vi "DisplacementTest.vi"() -> ()   [LabVIEW 2016]
uses:
  Displacement/DisplacementErrorCodes.ctl
  Telemetry/TelemetryFields.ctl
  <vilib>/rvi/Emulation/niFpgaGetClockAttributes.vi
  <vilib>/rvi/Emulation/niFpgaSctlEmulationGetInTimedLoop.vi
  <vilib>/rvi/Emulation/niFpgaEmulationReportErrorSimple.vi
  <vilib>/rvi/Emulation/niFpgaEmulationIsFPGAContextNoSignature.vi
  <vilib>/rvi/errors/niFpgaSetErrorForExecOnDevCompSimple.vi
  <vilib>/rvi/eio/common/nirviEmuReportErrorAndStop.vi
  <vilib>/rvi/DataTransferAndStorage/Container/Common/niFpgaContainerGetUniqueNameForEmu.vi
  <vilib>/rvi/FIFO/Fifo_Resource/nirvififoEmulationSetSize.vi
  <vilib>/rvi/FIFO/Fifo_Resource/nirviFifoEmulationQueueMgr.vi
  <instcachedir>/0/nirviFifoEmulationQueueMgr_E5CAEC123FF24DC58D834DCA3CDAA9B5.lvgen/nirviFifoEmulationQueueMgr_E5CAEC123FF24DC58D834DCA3CDAA9B5_004.vi
  <vilib>/rvi/FIFO/Fifo_Resource/nirvififoEmulationDetermineInputValidOut.vi
  <vilib>/rvi/FIFO/Fifo_Resource/nirvififoEmulationCreateLock.vi
  <vilib>/rvi/Emulation/niFpgaProcessEmulError.vi
  <vilib>/rvi/FIFO/Fifo_Resource/nirvififoEmulationObtainLock.vi
  <vilib>/rvi/FIFO/Fifo_Resource/nirvififoEmulationReleaseLock.vi
  <vilib>/rvi/occurrence/nirviWaitOnOccurrenceBase.vi
  <vilib>/rvi/errors/nirviReportUnexpectedCaseInternalError.vi
  <vilib>/rvi/errors/nirviReportUnexpectedCaseInternalError (U32).vi
  <vilib>/Utility/error.llb/Clear Errors.vi
  <vilib>/rvi/Emulation/niFpgaCriticalErrorInLSC.vi
  <vilib>/rvi/Memory/Memory_Emulation/nirvimemoryFastEmulation.vi
  <vilib>/rvi/Memory/Memory_Emulation/nirvimemoryEmulation.vi
  <vilib>/rvi/DataTransferAndStorage/Container/Common/niFpgaContainerExecOnDevCompGetState.vi
  <vilib>/rvi/Memory/Memory_Emulation/niFpgaMemoryEmulationCacheClearOnFirstRun.vi
  <vilib>/rvi/Memory/Memory_Emulation/nirvimemoryEmulationManagerCache_MakeExclusive.vi
  <vilib>/rvi/Memory/Memory_Emulation/niFpgaMemoryEmulationValidateCache.vi
  <vilib>/rvi/Memory/Memory_Emulation/nirvimemoryEmulationManagerCache_InsertValue.vi
  <vilib>/rvi/Memory/Memory_Emulation/nirvimemoryEmulationManagerCache_ReleaseExclusive.vi
  <vilib>/rvi/Memory/Memory_Emulation/nirvimemoryEmulationManagerCache_GetValue.vi
  <vilib>/rvi/Memory/Memory_Emulation/nirvimemoryEmulationManagerCache_SetValue.vi
  <vilib>/rvi/Emulation/niFpgaSctlEmulationResourceMgr.vi
  <instcachedir>/0/nirviFifoEmulationQueueMgr_E5CAEC123FF24DC58D834DCA3CDAA9B5.lvgen/nirviFifoEmulationQueueMgr_E5CAEC123FF24DC58D834DCA3CDAA9B5_035.vi
  <instcachedir>/0/nirviFifoEmulationQueueMgr_E5CAEC123FF24DC58D834DCA3CDAA9B5.lvgen/nirviFifoEmulationQueueMgr_E5CAEC123FF24DC58D834DCA3CDAA9B5_033.vi
  <instcachedir>/0/nirviFifoEmulationQueueMgr_E5CAEC123FF24DC58D834DCA3CDAA9B5.lvgen/nirviFifoEmulationQueueMgr_E5CAEC123FF24DC58D834DCA3CDAA9B5_030.vi
  <instcachedir>/0/nirviFifoEmulationQueueMgr_E5CAEC123FF24DC58D834DCA3CDAA9B5.lvgen/nirviFifoEmulationQueueMgr_E5CAEC123FF24DC58D834DCA3CDAA9B5_031.vi
  <vilib>/rvi/DataTransferAndStorage/Container/XNode/niFpgaContainer.xnode
  <vilib>/rvi/FIFO/Fifo_Resource/nirvififoEmulationWrite.vi
  <vilib>/rvi/FIFO/Fifo_Resource/nirvififoEmulationRead.vi
  <vilib>/rvi/Memory/Memory_Emulation/niFpgaMemoryEmulationRefIn.vi
panel:
  out "RotationZ":sgl
  out "RotationY":sgl
  out "RotationX":sgl
  out "PositionZ":sgl
  out "PositionY":sgl
  out "PositionX":sgl
  out "Eng8":sgl
  out "Eng7":sgl
  out "Eng6":sgl
  out "Eng5":sgl
  out "Eng4":sgl
  out "Eng3":sgl
  out "Eng2":sgl
  out "Raw8":i32
  out "Raw7":i32
  out "Raw6":i32
  out "Raw5":i32
  out "Raw4":i32
  out "Raw3":i32
  out "Raw2":i32
  out "Raw1":i32
  out "TxFrames":u64
  out "RxBytes":u64
  out "TxBytes":u64
  out "ErrorCode":T1
  out "ErrorTimestamp":u64
  out "RxFrames":u64
  out "Eng1":sgl
  out "SampleTimestamp":u64
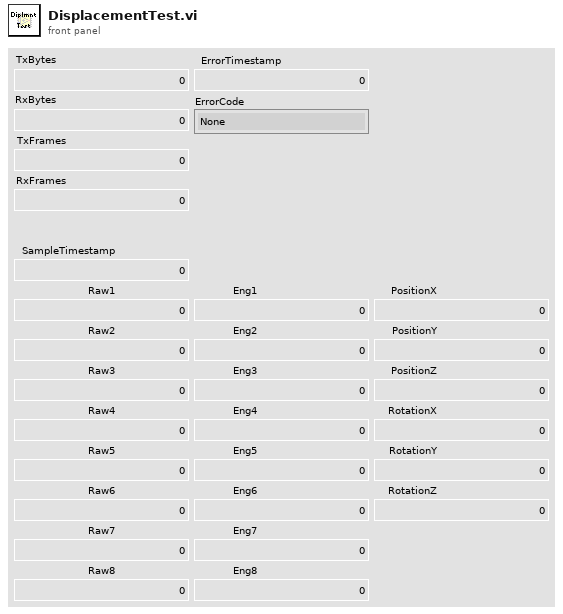
[diagram p1: front panel]
types:
  T1 = typedef "DisplacementErrorCodes.ctl" = enum16{"None", "ResponseUnknownError", "ResponseInvalidError", "ResponseTimeoutError", "SensorIndicatesInvalidCommandError", "SensorIndicatesCommunicationTimeoutError", "SensorIndicatesDataLengthError", "SensorIndicatesNumberOfParametersError", "SensorIndicatesParameterError", "SensorIndicatesCommunicationError", "SensorIndicatesIDNumberError", "SensorIndicatesExpansionLineError", "SensorIndicatesWriteControlError"}
  T2 = cluster{"Timestamp":u64, "TxBytes":u64, "RxBytes":u64, "TxFrames":u64, "RxFrames":u64, "RawAngle":i32, "ZenithAngle":sgl}
  T3 = cluster{"Timestamp":u64, "TxBytes":u64, "RxBytes":u64, "TxFrames":u64, "RxFrames":u64, "ErrorCode":enum8{"None", "ResponseAddressError", "ResponseFunctionCodeError", "ResponseByteCountError", "ResponseCRCError", "ResponseUnknownError", "ResponseTimeoutError", "SensorReportsIllegalFunction", "SensorReportsIllegalDataAddress"}}
  T4 = typedef "TelemetryFields.ctl" = enum16{"None", "InclinometerTxBytes", "InclinometerRxBytes", "InclinometerTxFrames", "InclinometerRxFrames", "InclinometerErrorTimestamp", "InclinometerErrorCode", "InclinometerSampleTimestamp", "InclinometerRawAngle", "InclinometerZenithAngle", "DisplacementTxBytes", "DisplacementRxBytes", "DisplacementTxFrames", "DisplacementRxFrames", "DisplacementErrorTimestamp", "DisplacementErrorCode", "DisplacementSampleTimestamp", "DisplacementRaw1", "DisplacementRaw2", "DisplacementRaw3", "DisplacementRaw4", "DisplacementRaw5", "DisplacementRaw6", "DisplacementRaw7", "DisplacementRaw8", "DisplacementEng1", "DisplacementEng2", "DisplacementEng3", "DisplacementEng4", "DisplacementEng5", "DisplacementEng6", "DisplacementEng7", "DisplacementEng8", "DisplacementPositionX", "DisplacementPositionY", "DisplacementPositionZ", "DisplacementRotationX", "DisplacementRotationY", "DisplacementRotationZ", "AccelerometerSampleCount", "AccelerometerTimestamp", "AccelerometerRaw1", "AccelerometerRaw2", "AccelerometerRaw3", "AccelerometerRaw4", "AccelerometerRaw5", "AccelerometerRaw6", "AccelerometerRaw7", "AccelerometerRaw8", "AccelerometerEng1", "AccelerometerEng2", "AccelerometerEng3", "AccelerometerEng4", "AccelerometerEng5", "AccelerometerEng6", "AccelerometerEng7", "AccelerometerEng8", "AngularAccelerationX", "AngularAccelerationY", "AngularAccelerationZ"}
diagram:
  n1 = while {
    stop <- FALSE stop-if-true
    n2 = flat-sequence {
      frame #0 {
        n3 = call "Loop Timer"("Count(mSec)"=u32 40) -> ()  [unwired: 1 out]
      }
      frame #1 {
        n4 = xnode ("FIFO Method Node")("Element"=TRUE, "Timeout"=0) -> ()  [unwired: 1 in, 2 out]
      }
      frame #2 {
        n5 = xnode ("FIFO Method Node")("Timeout"=-1) -> ()  [unwired: 1 in, 3 out]
      }
      frame #3 {
        n6 = call "TelemetryFieldToAddress.vi"("TelemetryFields"=TelemetryFields."DisplacementTxBytes") -> ("Address"=w32:u32)  [unwired: 10 in]
        n7 = call "ReadU64.vi"("Address"=w32) -> ("Data"=→"TxBytes":u64)  [unwired: 10 in]
      }
      frame #4 {
        n8 = call "TelemetryFieldToAddress.vi"("TelemetryFields"=TelemetryFields."DisplacementRxBytes") -> ("Address"=w37:u32)  [unwired: 10 in]
        n9 = call "ReadU64.vi"("Address"=w37) -> ("Data"=→"RxBytes":u64)  [unwired: 10 in]
      }
      frame #5 {
        n10 = call "TelemetryFieldToAddress.vi"("TelemetryFields"=TelemetryFields."DisplacementTxFrames") -> ("Address"=w38:u32)  [unwired: 10 in]
        n11 = call "ReadU64.vi"("Address"=w38) -> ("Data"=→"TxFrames":u64)  [unwired: 10 in]
      }
      frame #6 {
        n12 = call "TelemetryFieldToAddress.vi"("TelemetryFields"=TelemetryFields."DisplacementRxFrames") -> ("Address"=w43:u32)  [unwired: 10 in]
        n13 = call "ReadU64.vi"("Address"=w43) -> ("Data"=→"RxFrames":u64)  [unwired: 10 in]
      }
      frame #7 {
        n14 = call "TelemetryFieldToAddress.vi"("TelemetryFields"=TelemetryFields."DisplacementSampleTimestamp") -> ("Address"=w46:u32)  [unwired: 10 in]
        n15 = call "ReadU64.vi"("Address"=w46) -> ("Data"=→"SampleTimestamp":u64)  [unwired: 10 in]
      }
      frame #8 {
        n16 = call "TelemetryFieldToAddress.vi"("TelemetryFields"=TelemetryFields."DisplacementRaw1") -> ("Address"=w47:u32)  [unwired: 10 in]
        n17 = call "ReadI32.vi"("Address"=w47) -> ("Data"=→"Raw1":i32)  [unwired: 10 in]
      }
      frame #9 {
        n18 = call "TelemetryFieldToAddress.vi"("TelemetryFields"=TelemetryFields."DisplacementRaw2") -> ("Address"=w52:u32)  [unwired: 10 in]
        n19 = call "ReadI32.vi"("Address"=w52) -> ("Data"=→"Raw2":i32)  [unwired: 10 in]
      }
      frame #10 {
        n20 = call "TelemetryFieldToAddress.vi"("TelemetryFields"=TelemetryFields."DisplacementRaw3") -> ("Address"=w53:u32)  [unwired: 10 in]
        n21 = call "ReadI32.vi"("Address"=w53) -> ("Data"=→"Raw3":i32)  [unwired: 10 in]
      }
      frame #11 {
        n22 = call "TelemetryFieldToAddress.vi"("TelemetryFields"=TelemetryFields."DisplacementRaw4") -> ("Address"=w58:u32)  [unwired: 10 in]
        n23 = call "ReadI32.vi"("Address"=w58) -> ("Data"=→"Raw4":i32)  [unwired: 10 in]
      }
      frame #12 {
        n24 = call "TelemetryFieldToAddress.vi"("TelemetryFields"=TelemetryFields."DisplacementRaw5") -> ("Address"=w59:u32)  [unwired: 10 in]
        n25 = call "ReadI32.vi"("Address"=w59) -> ("Data"=→"Raw5":i32)  [unwired: 10 in]
      }
      frame #13 {
        n26 = call "TelemetryFieldToAddress.vi"("TelemetryFields"=TelemetryFields."DisplacementRaw6") -> ("Address"=w64:u32)  [unwired: 10 in]
        n27 = call "ReadI32.vi"("Address"=w64) -> ("Data"=→"Raw6":i32)  [unwired: 10 in]
      }
      frame #14 {
        n28 = call "TelemetryFieldToAddress.vi"("TelemetryFields"=TelemetryFields."DisplacementRaw7") -> ("Address"=w65:u32)  [unwired: 10 in]
        n29 = call "ReadI32.vi"("Address"=w65) -> ("Data"=→"Raw7":i32)  [unwired: 10 in]
      }
      frame #15 {
        n30 = call "TelemetryFieldToAddress.vi"("TelemetryFields"=TelemetryFields."DisplacementRaw8") -> ("Address"=w70:u32)  [unwired: 10 in]
        n31 = call "ReadI32.vi"("Address"=w70) -> ("Data"=→"Raw8":i32)  [unwired: 10 in]
      }
      frame #16 {
        n32 = call "TelemetryFieldToAddress.vi"("TelemetryFields"=TelemetryFields."DisplacementEng1") -> ("Address"=w73:u32)  [unwired: 10 in]
        n33 = call "ReadSGL.vi"("Address"=w73) -> ("Data"=→"Eng1":sgl)  [unwired: 10 in]
      }
      frame #17 {
        n34 = call "TelemetryFieldToAddress.vi"("TelemetryFields"=TelemetryFields."DisplacementEng2") -> ("Address"=w74:u32)  [unwired: 10 in]
        n35 = call "ReadSGL.vi"("Address"=w74) -> ("Data"=→"Eng2":sgl)  [unwired: 10 in]
      }
      frame #18 {
        n36 = call "TelemetryFieldToAddress.vi"("TelemetryFields"=TelemetryFields."DisplacementEng3") -> ("Address"=w79:u32)  [unwired: 10 in]
        n37 = call "ReadSGL.vi"("Address"=w79) -> ("Data"=→"Eng3":sgl)  [unwired: 10 in]
      }
      frame #19 {
        n38 = call "TelemetryFieldToAddress.vi"("TelemetryFields"=TelemetryFields."DisplacementEng4") -> ("Address"=w80:u32)  [unwired: 10 in]
        n39 = call "ReadSGL.vi"("Address"=w80) -> ("Data"=→"Eng4":sgl)  [unwired: 10 in]
      }
      frame #20 {
        n40 = call "TelemetryFieldToAddress.vi"("TelemetryFields"=TelemetryFields."DisplacementEng5") -> ("Address"=w85:u32)  [unwired: 10 in]
        n41 = call "ReadSGL.vi"("Address"=w85) -> ("Data"=→"Eng5":sgl)  [unwired: 10 in]
      }
      frame #21 {
        n42 = call "TelemetryFieldToAddress.vi"("TelemetryFields"=TelemetryFields."DisplacementEng6") -> ("Address"=w86:u32)  [unwired: 10 in]
        n43 = call "ReadSGL.vi"("Address"=w86) -> ("Data"=→"Eng6":sgl)  [unwired: 10 in]
      }
      frame #22 {
        n44 = call "TelemetryFieldToAddress.vi"("TelemetryFields"=TelemetryFields."DisplacementEng7") -> ("Address"=w91:u32)  [unwired: 10 in]
        n45 = call "ReadSGL.vi"("Address"=w91) -> ("Data"=→"Eng7":sgl)  [unwired: 10 in]
      }
      frame #23 {
        n46 = call "TelemetryFieldToAddress.vi"("TelemetryFields"=TelemetryFields."DisplacementEng8") -> ("Address"=w94:u32)  [unwired: 10 in]
        n47 = call "ReadSGL.vi"("Address"=w94) -> ("Data"=→"Eng8":sgl)  [unwired: 10 in]
      }
      frame #24 {
        n48 = call "TelemetryFieldToAddress.vi"("TelemetryFields"=TelemetryFields."DisplacementPositionX") -> ("Address"=w95:u32)  [unwired: 10 in]
        n49 = call "ReadSGL.vi"("Address"=w95) -> ("Data"=→"PositionX":sgl)  [unwired: 10 in]
      }
      frame #25 {
        n50 = call "TelemetryFieldToAddress.vi"("TelemetryFields"=TelemetryFields."DisplacementPositionY") -> ("Address"=w100:u32)  [unwired: 10 in]
        n51 = call "ReadSGL.vi"("Address"=w100) -> ("Data"=→"PositionY":sgl)  [unwired: 10 in]
      }
      frame #26 {
        n52 = call "TelemetryFieldToAddress.vi"("TelemetryFields"=TelemetryFields."DisplacementPositionZ") -> ("Address"=w101:u32)  [unwired: 10 in]
        n53 = call "ReadSGL.vi"("Address"=w101) -> ("Data"=→"PositionZ":sgl)  [unwired: 10 in]
      }
      frame #27 {
        n54 = call "TelemetryFieldToAddress.vi"("TelemetryFields"=TelemetryFields."DisplacementRotationX") -> ("Address"=w106:u32)  [unwired: 10 in]
        n55 = call "ReadSGL.vi"("Address"=w106) -> ("Data"=→"RotationX":sgl)  [unwired: 10 in]
      }
      frame #28 {
        n56 = call "TelemetryFieldToAddress.vi"("TelemetryFields"=TelemetryFields."DisplacementRotationY") -> ("Address"=w107:u32)  [unwired: 10 in]
        n57 = call "ReadSGL.vi"("Address"=w107) -> ("Data"=→"RotationY":sgl)  [unwired: 10 in]
      }
      frame #29 {
        n58 = call "TelemetryFieldToAddress.vi"("TelemetryFields"=TelemetryFields."DisplacementRotationZ") -> ("Address"=w112:u32)  [unwired: 10 in]
        n59 = call "ReadSGL.vi"("Address"=w112) -> ("Data"=→"RotationZ":sgl)  [unwired: 10 in]
      }
      frame #30 {
        n60 = call "TelemetryFieldToAddress.vi"("TelemetryFields"=TelemetryFields."DisplacementErrorTimestamp") -> ("Address"=w113:u32)  [unwired: 10 in]
        n61 = call "ReadU64.vi"("Address"=w113) -> ("Data"=→"ErrorTimestamp":u64)  [unwired: 10 in]
      }
      frame #31 {
        n62 = call "TelemetryFieldToAddress.vi"("TelemetryFields"=TelemetryFields."DisplacementErrorCode") -> ("Address"=w117:u32)  [unwired: 10 in]
        n63 = call "ReadU8.vi"("Address"=w117) -> ("Data"=→"ErrorCode":u8)  [unwired: 10 in]
      }
      frame #32 {
        n64 = xnode ("FIFO Method Node")("Element"=TRUE, "Timeout"=0) -> ()  [unwired: 1 in, 2 out]
      }
    }
  }
  n65 = call "Displacement.vi"() -> ()  [unwired: 12 in]
  n66 = call "Telemetry.vi"() -> ()  [unwired: 12 in]
  n67 = xnode ("Memory Method Node")("Address"=u32 0, "Data"=sgl 1.0) -> ("Memory Out"=w20:refnum<k21>)  [unwired: 1 in]
  n68 = xnode ("FIFO Method Node")("Timeout"=0) -> ()  [unwired: 1 in, 3 out]
  n69 = xnode ("FIFO Method Node")("Element"=T2 {"Timestamp"=0, "TxBytes"=0, "RxBytes"=0, "TxFrames"=0, "RxFrames"=0, "RawAngle"=0, "ZenithAngle"=0.0}, "Timeout"=0) -> ()  [unwired: 1 in, 2 out]
  n70 = xnode ("FIFO Method Node")("Timeout"=0) -> ()  [unwired: 1 in, 3 out]
  n71 = xnode ("FIFO Method Node")("Element"=T3 {"Timestamp"=0, "TxBytes"=0, "RxBytes"=0, "TxFrames"=0, "RxFrames"=0, "ErrorCode"=enum."None"}, "Timeout"=0) -> ()  [unwired: 1 in, 2 out]
  n72 = xnode ("FIFO Method Node")("Timeout"=0) -> ()  [unwired: 1 in, 3 out]
  n73 = xnode ("Memory Method Node")("Address"=u32 9, "Data"=sgl 1.0, "Memory In"=w20) -> ("Memory Out"=w19:refnum<k21>)
  n74 = xnode ("Memory Method Node")("Address"=u32 18, "Data"=sgl 1.0, "Memory In"=w19) -> ("Memory Out"=w12:refnum<k21>)
  n75 = xnode ("FIFO Method Node")("Timeout"=0) -> ()  [unwired: 1 in, 3 out]
  n76 = xnode ("FIFO Method Node")("Timeout"=0) -> ()  [unwired: 1 in, 3 out]
  n77 = xnode ("Memory Method Node")("Address"=u32 27, "Data"=sgl 1.0, "Memory In"=w12) -> ("Memory Out"=w11:refnum<k21>)
  n78 = xnode ("Memory Method Node")("Address"=u32 36, "Data"=sgl 1.0, "Memory In"=w11) -> ("Memory Out"=w10:refnum<k21>)
  n79 = xnode ("Memory Method Node")("Address"=u32 45, "Data"=sgl 1.0, "Memory In"=w10) -> ()  [unwired: 1 out]
